vi "Config-Chan-GNDU.vi"(8 "error in (no error)":errorcluster, 9 "state":bool, 10 "V name \n(max 6 chars)":string, 11 "VISA session":refnum<visa-resource-name>) -> (0 "error out":errorcluster, 3 "VISA resource name out":refnum<visa-resource-name>)   [LabVIEW 2016, in "Agilent 415X Series.lvlib"]
doc: "This VI configures the GNDU in the Expander Unit (if installed).\n\n** The instrument used in the development of this instrument driver does not have an Expander Unit installed. Therefore commands related to GNDU have not been verified."
uses:
  Agilent 415X Series.lvlib
panel:
  # "* This VI has not been verified on\nan HP415xA with a GNDU.  \nPlease report problems to \n     National Instruments\n     1-800-IEEE488.\nThanks!"
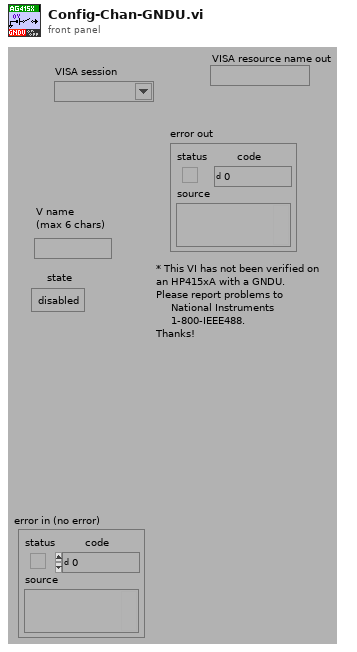
[diagram p1: front panel]
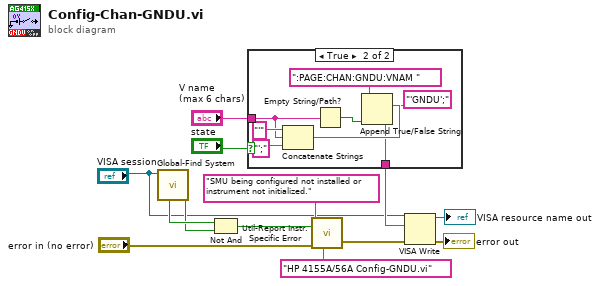
[diagram p0: block diagram]
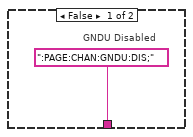
[diagram p2: hidden frame]
diagram:
  n1 = call "Global-Find System.vi"("VISA session"="VISA session") -> ("found"=w3:bool, "GNDU present"=w4:bool)  [unwired: 3 in, 6 out]
  n2 = Not And(1:w3, 2:w4) -> (0:w6:bool)
  n3 = case shown="True" "state" {
    tunnel: "V name \n(max 6 chars)" -> [_ w20]
    tunnel: [":PAGE:CHAN:GNDU:DIS;" w15] -> w11
    frame False {
      # "GNDU Disabled"
    }
    frame True {
      n4 = Concatenate Strings("'", w20, "';") -> (w19:string)
      n5 = Empty String/Path?(string/path=w20) -> (empty?=w22:bool)
      n6 = Append True/False String(1:w22, 2:w19, 3:"'GNDU';", 4:":PAGE:CHAN:GNDU:VNAM ") -> (0:w15:string)
    }
  }
  n7 = call "Util-Report Instr. Specific Error.vi"("source"="HP 4155A/56A Config-GNDU.vi", "error in (no error)"="error in (no error)", "error message"="SMU being configured not installed or instrument not initialized.", "new error"=w6) -> ("error out"=w9:errorcluster)  [unwired: 6 in, 1 out]
  n8 = VISA Write(VISA resource name="VISA session", write buffer=w11, error in (no error)=w9) -> (VISA resource name out=→"VISA resource name out":refnum<visa-resource-name>, error out=→"error out":errorcluster)  [unwired: 1 out]
